vi "注册接收数据已改变事件.vi"(8 "error in (no error)":errorcluster caption="错误输入（无错误）", 10 "Ctl引用句柄":refnum<vi>, 11 "串口 输入":refnum<class "串口.lvclass"> caption="DNL_LabVIEW Object in") -> (0 "error out":errorcluster caption="错误输出", 3 "串口 输出":refnum<class "串口.lvclass"> caption="DNL_LabVIEW Object out")   [LabVIEW 2012, in "串口.lvclass"]
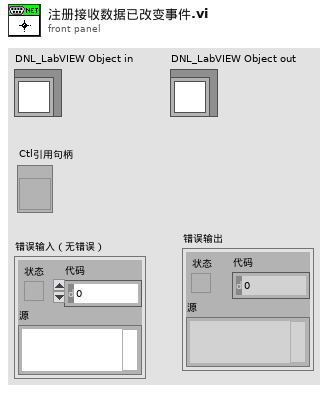
[diagram p1: front panel]
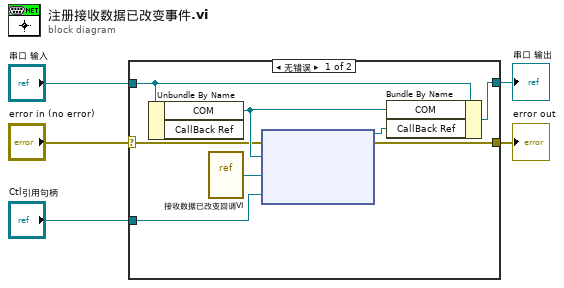
[diagram p0: block diagram]
diagram:
  n1 = case shown="无错误" "error in (no error)" {
    selector: "error in (no error)" -> [w7 w15]
    tunnel: [w6 w15] -> w4
    tunnel: [w8 w14] -> w2
    tunnel: "串口 输入" -> [w11 w14]
    tunnel: "Ctl引用句柄" -> [w13 _]
    frame No Error {
      n2 = Unbundle By Name(w11) -> ("COM"=w10:refnum<k24>)  [unwired: 1 out]
      n3 = vi-ref "接收数据已改变回调VI.vi"() -> ("vi reference"=w12:refnum<vi>)
      n4 = node(w7, w10, w12, w13) -> (w9:refnum<k27>, w6:errorcluster)  [unwired: 1 in]
      n5 = Bundle By Name(cluster=w11, "COM"=w10, "CallBack Ref"=w9) -> (w8:refnum<class "串口.lvclass">)
    }
    frame Error {
    }
  }
  "error out" <- w4
  "串口 输出" <- w2
